vi "Example Power Supply.vi"() -> ()   [LabVIEW 2015]
panel:
  out "Pos Read":dbl(slide) scale=0.0..5.0
  out "Neg Read":dbl(slide)
  in  "Stop Button":bool
  in  "Neg  V":dbl min=-5.0 max=0.0
  in  "Pos V":dbl min=0.0 max=5.0
  in  "Positive channel":bool
  in  "Negative channel":bool
  in  "Calibrate":bool
  in  "Active ADALM2000 URIs:":u16(ring) items=["ip:192.168.2.1", "usb:2.9.5", "usb:2.9.5"]
  in  "Connect Btn":bool
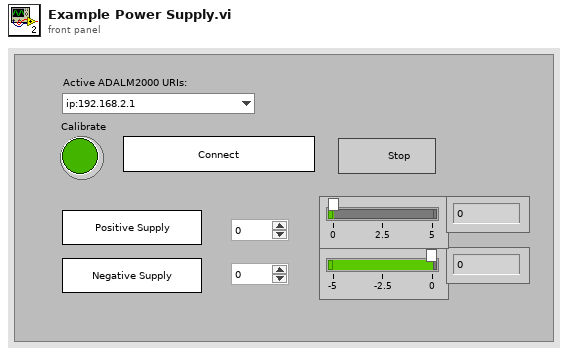
[diagram p1: front panel]
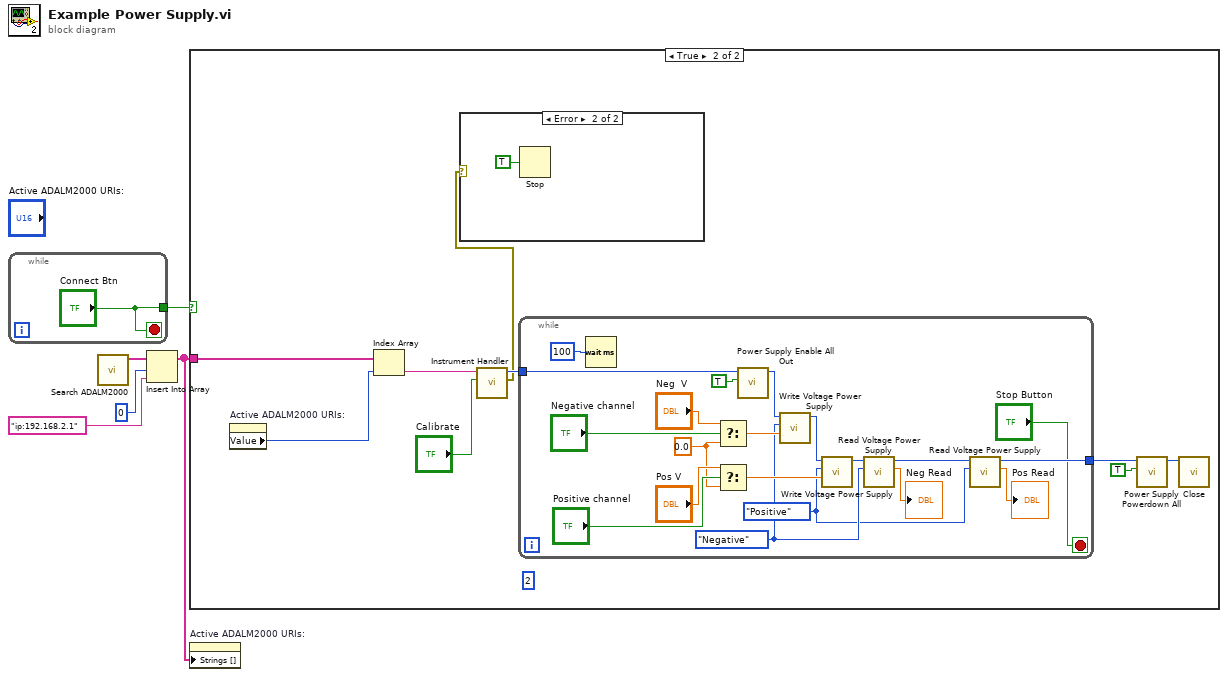
[diagram p0: block diagram]
diagram:
  n1 = while {
    tunnel: ["Connect Btn"] -> w2
    stop <- "Connect Btn" stop-if-true
  }
  n2 = call "Search ADALM2000.vi"() -> ("Array"=w5:string[])  [unwired: 11 in]
  n3 = Insert Into Array(array=w5, index=0, new element="ip:192.168.2.1" ("new element/subarray")) -> (w1:string[])
  n4 = case shown="True" w2 {
    tunnel: w1 -> [_ w14]
    frame False {
    }
    frame True {
      (unwired) 2
      n5 = property on="Active ADALM2000 URIs:" class="Ring (strict)"() -> ("Value"=w13:u16)  [unwired: 2 in, 2 out]
      n6 = Index Array(array=w14, index=w13) -> (element=w12:string)
      n7 = call "Instrument Handler.vi"("Calibrate"="Calibrate", "ADALM2000 URI"=w12) -> ("error out"=w7:errorcluster, "ADALM2000 Handle"=w10:u32)  [unwired: 8 in]
      n8 = case shown="Error" w7 {
        frame No Error {
        }
        frame Error {
          n9 = Stop(stop? (T)=TRUE) -> ()
        }
      }
      n10 = while {
        tunnel: w10 -> [w36]
        tunnel: [w35] -> w9
        stop <- "Stop Button" stop-if-true
        w23 = enum16{"Positive", "Negative"}."Negative" ("Channel")
        w21 = enum16{"Positive", "Negative"}."Positive" ("Channel")
        w28 = 0.0 ("f")
        n11 = Wait (ms)(milliseconds to wait=u32 100) -> ()  [unwired: 1 out]
        n12 = Select(t="Neg  V", s="Negative channel", f=w28) -> (s? t:f=w26:dbl)
        n13 = Select(t="Pos V", s="Positive channel", f=w28) -> (s? t:f=w27:dbl)
        n14 = call "Power Supply Enable All Out.vi"("Enable"=TRUE, "ADALM2000 Handler"=w36) -> ("ADALM2000 Handler 2"=w20:u32)  [unwired: 9 in]
        n15 = call "Write Voltage Power Supply.vi"("Voltage"=w26, "Channel"=w23, "ADALM2000 Handler"=w20) -> ("ADALM2000 Handler 2"=w25:u32)  [unwired: 8 in]
        n16 = call "Write Voltage Power Supply.vi"("Voltage"=w27, "Channel"=w21, "ADALM2000 Handler"=w25) -> ("ADALM2000 Handler 2"=w24:u32)  [unwired: 8 in]
        n17 = call "Read Voltage Power Supply.vi"("Channel"=w23, "ADALM2000 Handler"=w24) -> ("Read Voltage"=→"Neg Read":dbl, "ADALM2000 Handler 2"=w22:u32)  [unwired: 8 in]
        n18 = call "Read Voltage Power Supply.vi"("Channel"=w21, "ADALM2000 Handler"=w22) -> ("Read Voltage"=→"Pos Read":dbl, "ADALM2000 Handler 2"=w35:u32)  [unwired: 8 in]
      }
      n19 = call "Power Supply Powerdown All.vi"("Powerdown"=TRUE, "ADALM2000 Handler"=w9) -> ("ADALM2000 Handler 2"=w15:u32)  [unwired: 9 in]
      n20 = call "Close.vi"("ADALM2000 Handler"=w15) -> ()  [unwired: 11 in]
    }
  }
  n21 = property on="Active ADALM2000 URIs:" class="Ring (strict)"("Strings []"=w1) -> ()  [unwired: 2 in, 2 out]
